vi "write array value to Ref.vi"(8 "error in (no error)":errorcluster, 10 "Value":refnum<class "Generic Instrument.lvclass">[](array[class]), 11 "Controller.lvclass":refnum<class "Controller.lvclass">) -> (0 "error out":errorcluster, 3 "Controller out":refnum<class "Controller.lvclass">)   [LabVIEW 2014, in "Controller.lvclass"]
uses:
  Controller.lvclass
  Generic Instrument/Generic Instrument.lvclass
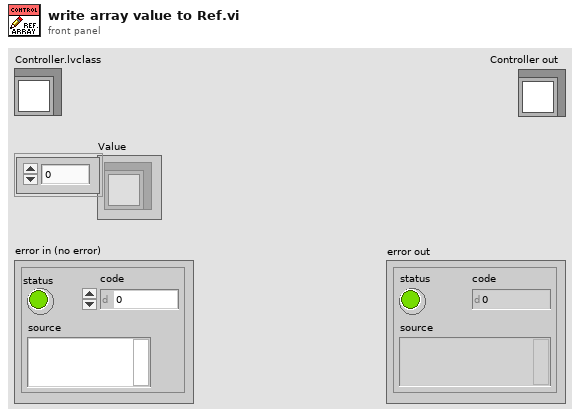
[diagram p1: front panel]
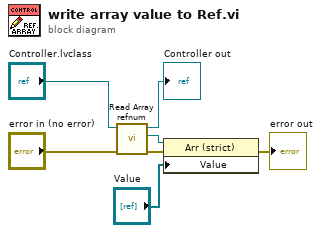
[diagram p0: block diagram]
diagram:
  n1 = call-dynamic "Read Array refnum.vi"("error in (no error)"="error in (no error)", "Controller in"="Controller.lvclass") -> ("error out"=w4:errorcluster, "Array refnum"=w6:refnum<vi>, "Controller out"=→"Controller out":refnum<class "Controller.lvclass">)  [unwired: 7 in]
  n2 = property class="Arr (strict)"(reference=w6, error in=w4, "Value"="Value") -> (error out=→"error out":errorcluster)  [unwired: 1 out]
